vi "Database.UpdateVariantFilesss.vi"(8 "error in (no error)":errorcluster, 11 "Data in":T1 {"Variant"."TS"."TV"."minimum" format="%#.3f"; "Variant"."TS"."TV"."maximum" format="%#.3f"; "Variant"."TS"."TP"."value" format="%#.3f"}) -> (0 "error out":errorcluster, 3 "Data out":T1 {"Variant"."TS"."TV"."minimum" format="%#.3f"; "Variant"."TS"."TV"."maximum" format="%#.3f"; "Variant"."TS"."TP"."value" format="%#.3f"})   [LabVIEW 2016]
uses:
  Database.Main.Data.ctl
  Database.Main.Data.Status.ctl
  Database.Main.Data.Sets.ctl
  Database.Main.Data.Results.ctl
  ProdaNG/Controls/ProdaNG.Identification.ctl
  ProdaNG/Controls/ProdaNG.ProcessResult.ctl
  ProdaNG/Controls/ProdaNG.ProcessStepResult.ctl
  ProdaNG/Controls/ProdaNG.TestStepResult.ctl
  ProdaNG/Controls/ProdaNG.TestValueResult.ctl
  Database.Main.Data.Variant.ctl
  ProdaNG/Controls/ProdaNG.ProcessStepParam.ctl
  ProdaNG/Controls/ProdaNG.TestStep.ctl
  ProdaNG/Controls/ProdaNG.TestStepParam.ctl
  ProdaNG/Controls/ProdaNG.TestValue.ctl
  Global/ApplicationGlobal.vi
panel:
  out "output 1":timestamp
  out "LatestChange":timestamp
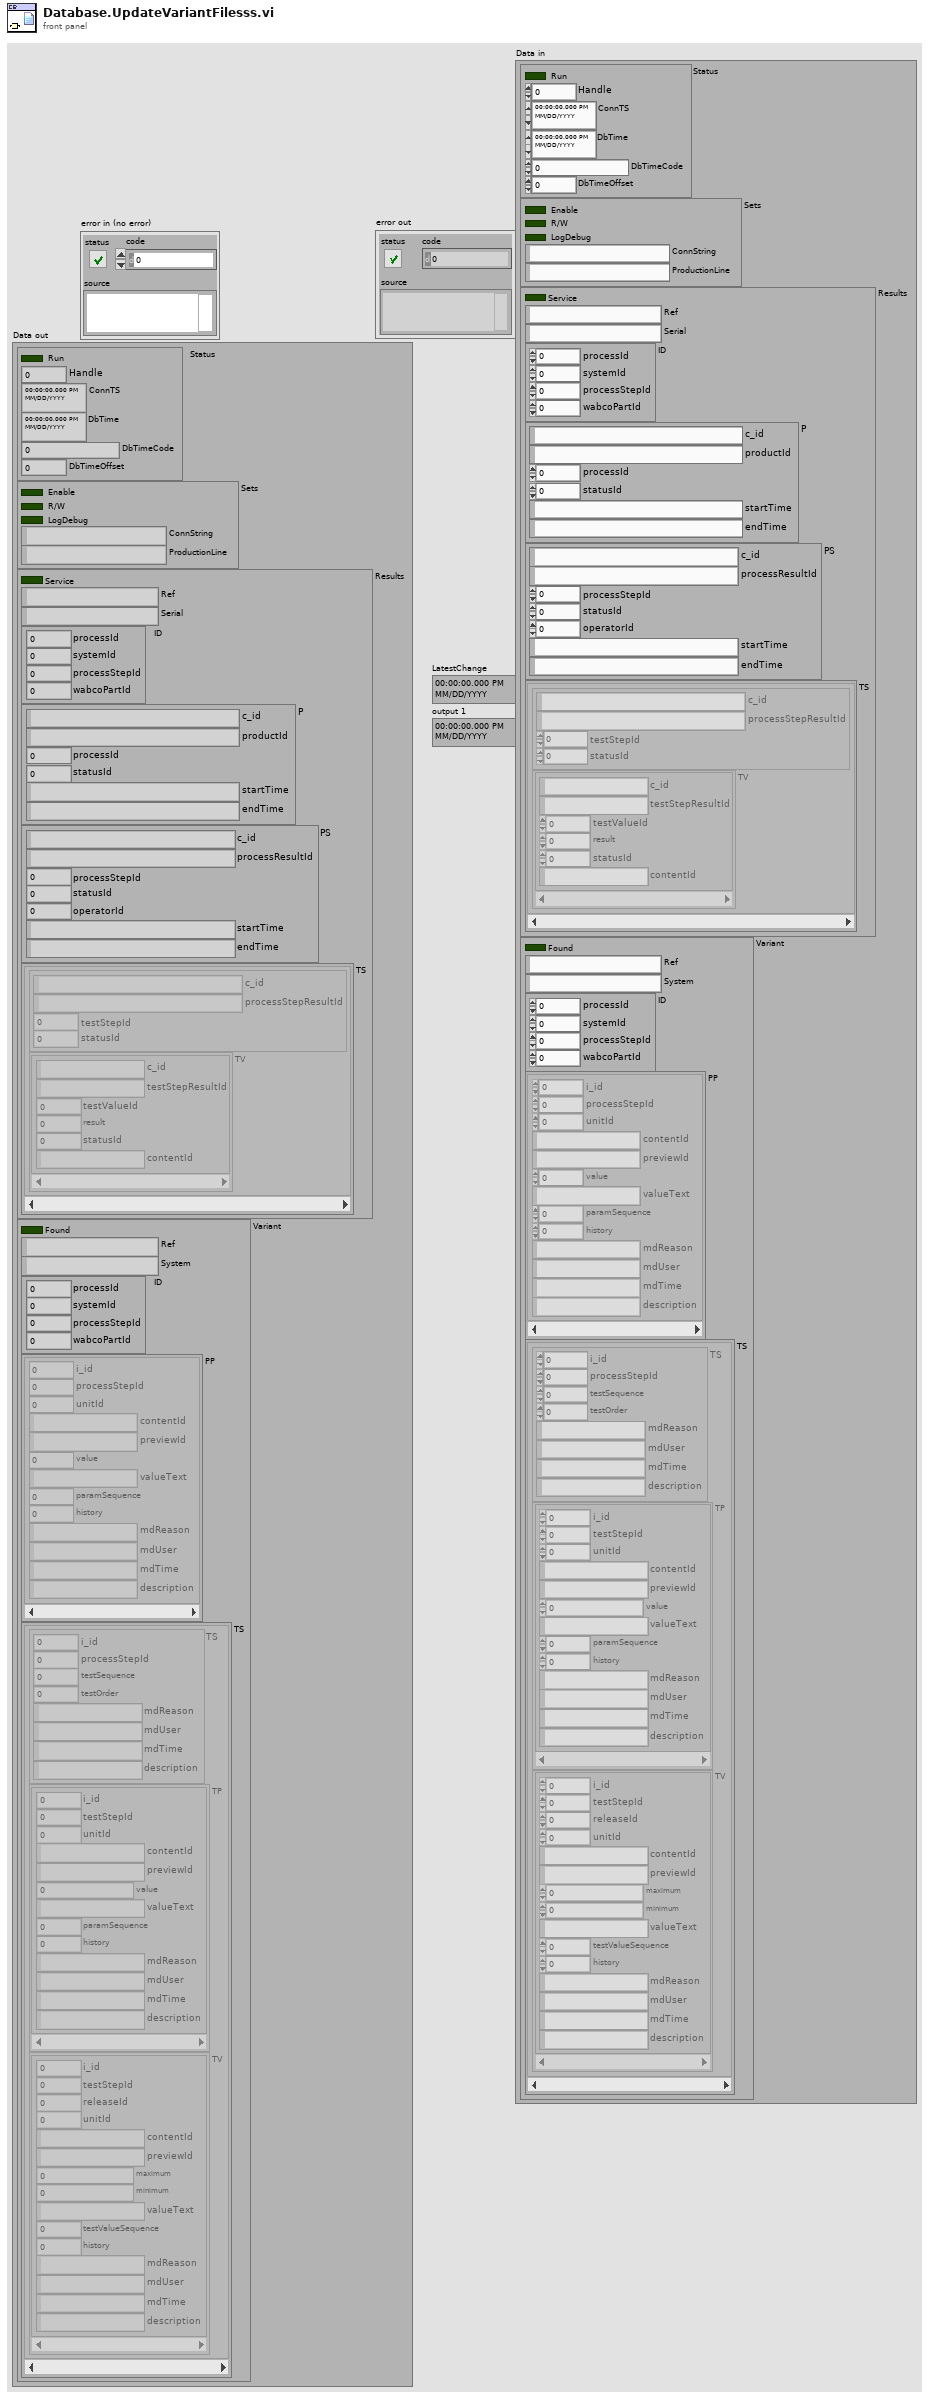
[diagram p1: front panel]
types:
  T1 = typedef "Database.Main.Data.ctl" = cluster{"Status":T2, "Sets":T3, "Results":T4, "Variant":T10}
  T2 = typedef "Database.Main.Data.Status.ctl" = cluster{"Run":bool, "Handle":i32, "ConnTS":timestamp, "DbTime":timestamp, "DbTimeCode":dbl, "DbTimeOffset":dbl}
  T3 = typedef "Database.Main.Data.Sets.ctl" = cluster{"Enable":bool, "R/W":bool, "LogDebug":bool, "ConnString":string, "ProductionLine":string}
  T4 = typedef "Database.Main.Data.Results.ctl" = cluster{"Service":bool, "Ref":string, "Serial":string, "ID":T5, "P":T6, "PS":T7, "TS":cluster{"TS":T8, "TV":T9[]}[]}
  T5 = typedef "ProdaNG.Identification.ctl" = cluster{"processId":i32, "systemId":i32, "processStepId":i32, "wabcoPartId":i32}
  T6 = typedef "ProdaNG.ProcessResult.ctl" = cluster{"c_id":string, "productId":string, "processId":i32, "statusId":i32, "startTime":string, "endTime":string}
  T7 = typedef "ProdaNG.ProcessStepResult.ctl" = cluster{"c_id":string, "processResultId":string, "processStepId":i32, "statusId":i32, "operatorId":i32, "startTime":string, "endTime":string}
  T8 = typedef "ProdaNG.TestStepResult.ctl" = cluster{"c_id":string, "processStepResultId":string, "testStepId":i32, "statusId":i32}
  T9 = typedef "ProdaNG.TestValueResult.ctl" = cluster{"c_id":string, "testStepResultId":string, "testValueId":i32, "result":dbl, "statusId":i32, "contentId":string}
  T10 = typedef "Database.Main.Data.Variant.ctl" = cluster{"Found":bool, "Ref":string, "System":string, "ID":T5, "PP":T11[], "TS":cluster{"TS":T12, "TP":T13[], "TV":T14[]}[]}
  T11 = typedef "ProdaNG.ProcessStepParam.ctl" = cluster{"i_id":i32, "processStepId":i32, "unitId":i32, "contentId":string, "previewId":string, "value":dbl, "valueText":string, "paramSequence":i32, "history":i32, "mdReason":string, "mdUser":string, "mdTime":string, "description":string}
  T12 = typedef "ProdaNG.TestStep.ctl" = cluster{"i_id":i32, "processStepId":i32, "testSequence":i32, "testOrder":i32, "mdReason":string, "mdUser":string, "mdTime":string, "description":string}
  T13 = typedef "ProdaNG.TestStepParam.ctl" = cluster{"i_id":i32, "testStepId":i32, "unitId":i32, "contentId":string, "previewId":string, "value":dbl, "valueText":string, "paramSequence":i32, "history":i32, "mdReason":string, "mdUser":string, "mdTime":string, "description":string}
  T14 = typedef "ProdaNG.TestValue.ctl" = cluster{"i_id":i32, "testStepId":i32, "releaseId":i32, "unitId":i32, "contentId":string, "previewId":string, "maximum":dbl, "minimum":dbl, "valueText":string, "testValueSequence":i32, "history":i32, "mdReason":string, "mdUser":string, "mdTime":string, "description":string}
  T15 = enum16{"open", "replace", "create", "open or create", "replace or create", "replace or create with confirmation"}
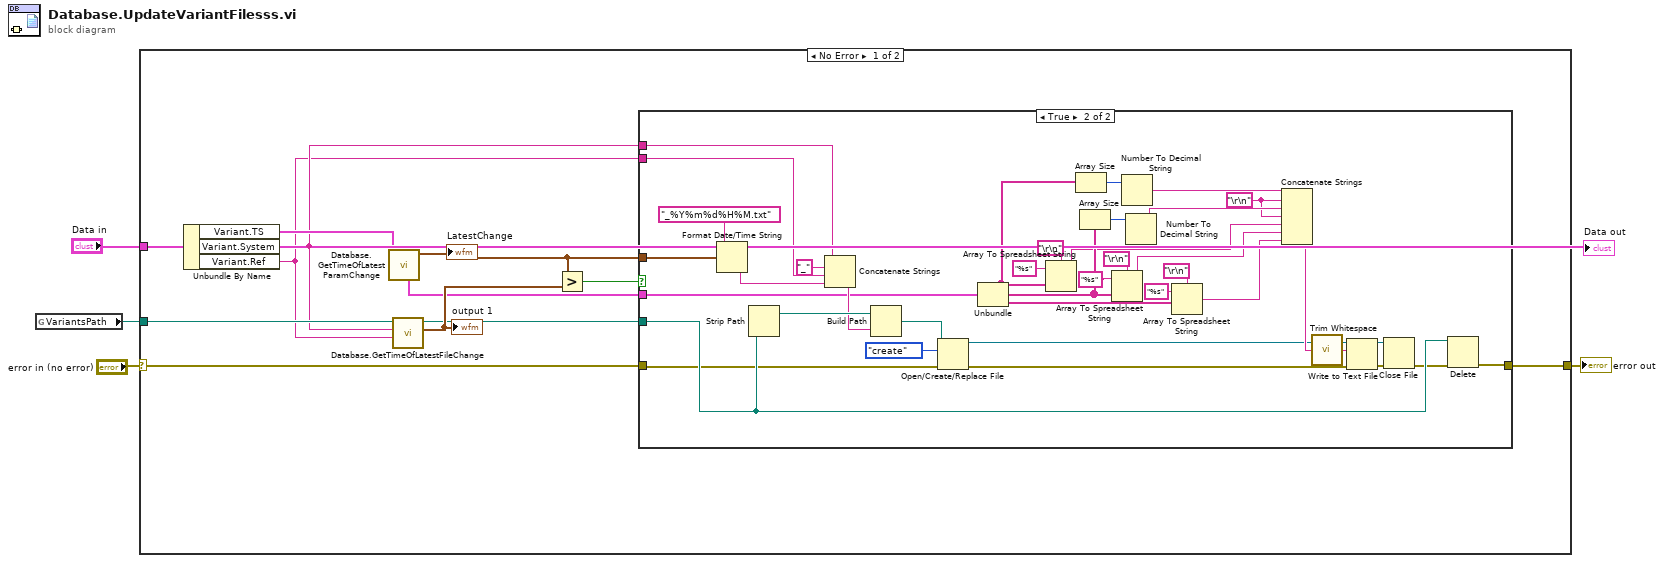
[diagram p0: block diagram]
diagram:
  n1 = global read "ApplicationGlobal.vi" "VariantsPath"() -> (w3:path)
  n2 = case shown="No Error" "error in (no error)" {
    selector: "error in (no error)" -> [w10 w56]
    tunnel: w3 -> [w14 _]
    tunnel: "Data in" -> [w16 _]
    tunnel: [w5 w56] -> w2
    frame No Error {
      n3 = Unbundle By Name(w16) -> ("Variant.TS"=w15:cluster{"TS":T12, "TP":T13[], "TV":T14[]}[], "Variant.System"=w8:string, "Variant.Ref"=w7:string)
      n4 = call "Database.GetTimeOfLatestParamChange.vi"("TS"=w15) -> ("Max"=w9:timestamp, "VariantFileValues"=w6:cluster{string[], string[], string[]})  [unwired: 6 in, 3 out]
      "LatestChange" <- w9
      n5 = call "Database.GetTimeOfLatestFileChange.vi"("Ref"=w7, "System"=w8, "VariantsFolder"=w14) -> ("Time Stamp"=w12:timestamp, "FilePath"=w11:path)  [unwired: 7 in]
      "output 1" <- w12
      n6 = Greater?(x=w9, y=w12) -> (0:w13:bool)
      n7 = case shown="True" w13 {
        tunnel: w11 -> [_ w54]
        tunnel: w10 -> [w17 w18]
        tunnel: w9 -> [_ w52]
        tunnel: w8 -> [_ w51]
        tunnel: w7 -> [_ w49]
        tunnel: w6 -> [_ w43]
        tunnel: [w17 w19] -> w5
        frame False {
        }
        frame True {
          w28 = "\r\n"
          n8 = Format Date/Time String(time format string (%c)="_%Y%m%d%H%M.txt" ("format string"), seconds (now)=w52) -> (date/time string=w48:string)  [unwired: 1 in]
          n9 = Strip Path(path=w54) -> (stripped path=w47:path)  [unwired: 1 out]
          n10 = Concatenate Strings(w51, "_" ("string"), w49, w48) -> (w46:string)
          n11 = Build Path(base path=w47, name or relative path=w46) -> (appended path=w45:path)
          n12 = Open/Create/Replace File(file path (use dialog)=w45, error in=w18, operation (0:open)=T15."create") -> (refnum out=w23:refnum<file>, error out=w44:errorcluster)  [unwired: 3 in, 1 out]
          n13 = Unbundle(w43) -> (w40:string[], w33:string[], w34:string[])
          n14 = Array To Spreadsheet String(delimiter (Tab)="\r\n", array=w40, 3:"%s" ("format string")) -> (spreadsheet string=w29:string)
          n15 = Array Size(array=w40) -> (size(s)=w39:i32)
          n16 = Array Size(array=w33) -> (size(s)=w32:i32)
          n17 = Array To Spreadsheet String(delimiter (Tab)="\r\n", array=w33, 3:"%s" ("format string")) -> (spreadsheet string=w22:string)
          n18 = Number To Decimal String(number=w39) -> (decimal integer string=w31:string)  [unwired: 1 in]
          n19 = Number To Decimal String(number=w32) -> (decimal integer string=w30:string)  [unwired: 1 in]
          n20 = Array To Spreadsheet String(delimiter (Tab)="\r\n", array=w34, 3:"%s" ("format string")) -> (spreadsheet string=w27:string)
          n21 = Concatenate Strings(w31, w28, w30, w28, w29, w22, w27) -> (w26:string)
          n22 = call <vilib>:"Trim Whitespace.vi"("string"=w26) -> ("trimmed string"=w21:string)  [unwired: 1 in]
          n23 = Write to Text File(file (use dialog)=w23, text=w21, error in=w44) -> (refnum out=w24:refnum<file>, error out=w25:errorcluster)  [unwired: 1 in, 1 out]
          n24 = Close File(refnum=w24, error in=w25) -> (error out=w20:errorcluster)  [unwired: 1 out]
          n25 = Delete(path (use dialog)=w54, error in=w20) -> (error out=w19:errorcluster)  [unwired: 3 in, 2 out]
        }
      }
    }
    frame Error {
    }
  }
  "error out" <- w2
  "Data out" <- "Data in"
